vi "Destructor.vi"(8 "error in":errorcluster, 11 "ProcessRun in":refnum<class "ProcessRun.lvclass">) -> (0 "error out":errorcluster)   [LabVIEW 2021, in "ProligentXMLGenerator.lvlib" / "ProcessRun.lvclass"]
uses:
  ProcessRun.lvclass
  ProcessRun.lvclass/ProcessRun.ctl
  OperationRun/OperationRun.lvclass
  OperationCycle/OperationCycle.lvclass
  Failure/FailureReference/FailureReference.lvclass
  Model/CustomData/CustomData.lvclass
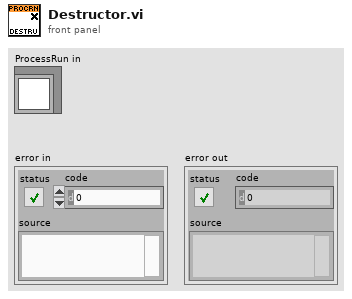
[diagram p1: front panel]
types:
  T1 = typedef "ProligentXMLGenerator.lvlib/ProcessRun.lvclass/Data.ctl" = cluster{"Name":string, "OperationRuns":refnum<class "OperationRun.lvclass">[], "OperationCycles":refnum<class "OperationCycle.lvclass">[], "FailureReferences":refnum<class "FailureReference.lvclass">[], "CustomData":refnum<class "CustomData.lvclass">, "ProcessRunId":refnum<class "Guid.lvclass">, "ProcessFullName":refnum<class "ProcessFullName.lvclass">, "ProcessVersion":refnum<class "NonEmptyString_64.lvclass">, "ProductUnitIdentifier":refnum<class "NonEmptyString_50.lvclass">, "ProductFullName":refnum<class "FullName.lvclass">, "ProcessRunStatus":refnum<class "ExecutionStatus.lvclass">, "ProcessRunStartTime":refnum<class "DateTime.lvclass">, "ProcessRunEndTime":refnum<class "DateTime.lvclass">, "ProcessMode":refnum<class "NonEmptyString_64.lvclass">, "TimeZoneInfoId":string}
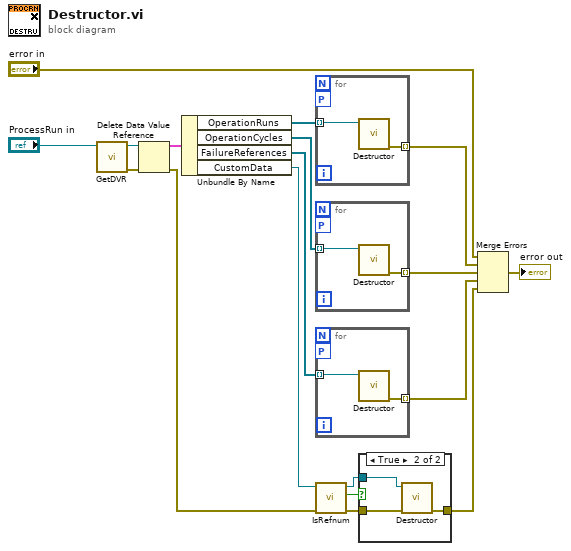
[diagram p0: block diagram]
diagram:
  n1 = call "GetDVR.vi"("ProcessRun"="ProcessRun in") -> ("error out"=w15:errorcluster, "DVRReference"=w16:refnum<data-value>)  [unwired: 9 in]
  n2 = Delete Data Value Reference(data value reference=w16, error in=w15) -> (data value=w14:T1, error out=w1:errorcluster)
  n3 = Unbundle By Name(w14) -> ("OperationRuns"=w11:refnum<class "OperationRun.lvclass">[], "OperationCycles"=w10:refnum<class "OperationCycle.lvclass">[], "FailureReferences"=w9:refnum<class "FailureReference.lvclass">[], "CustomData"=w3:refnum<class "CustomData.lvclass">)
  n4 = for {
    tunnel: w11 -> [w20] mode=indexing
    tunnel: [w19] -> w12 mode=indexing
    workers-P: _ -> [_]
    n5 = call "Destructor.vi"("OperationRun"=w20) -> ("error out"=w19:errorcluster)  [unwired: 10 in]
  }
  n6 = for {
    tunnel: w10 -> [w22] mode=indexing
    tunnel: [w21] -> w7 mode=indexing
    workers-P: _ -> [_]
    n7 = call "Destructor.vi"("OperationCycle in"=w22) -> ("error out"=w21:errorcluster)  [unwired: 10 in]
  }
  n8 = for {
    tunnel: w9 -> [w24] mode=indexing
    tunnel: [w23] -> w8 mode=indexing
    workers-P: _ -> [_]
    n9 = call "Destructor.vi"("FailureReference in"=w24) -> ("error out"=w23:errorcluster)  [unwired: 10 in]
  }
  n10 = call "IsRefnum.vi"("error in"=w1, "CustomDataType in"=w3) -> ("error out"=w4:errorcluster, "IsRefnum"=w6:bool, "CustomDataType out"=w5:refnum<class "CustomData.lvclass">)  [unwired: 7 in]
  n11 = case shown="True" w6 {
    tunnel: w5 -> [_ w28]
    tunnel: w4 -> [w25 w27]
    tunnel: [w25 w26] -> w2
    frame False {
    }
    frame True {
      n12 = call "Destructor.vi"("error in"=w27, "CustomDataType"=w28) -> ("error out"=w26:errorcluster)  [unwired: 9 in]
    }
  }
  n13 = Merge Errors("error in", w12, w7, w8, w2) -> (→"error out":errorcluster)
